vi "File taratura assente.vi"(8 "Curva 3":string[][](array[string]), 9 "Curva 2":string[][](array[string]), 10 "Curva 1":string[][](array[string]), 11 "P2":i32) -> (2 "File taratura assente":bool)   [LabVIEW 2019]
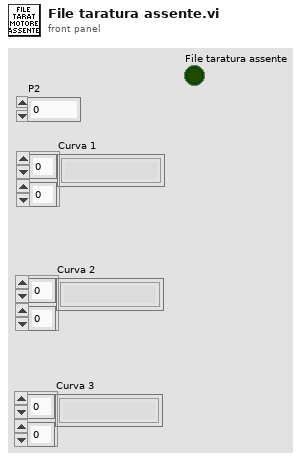
[diagram p1: front panel]
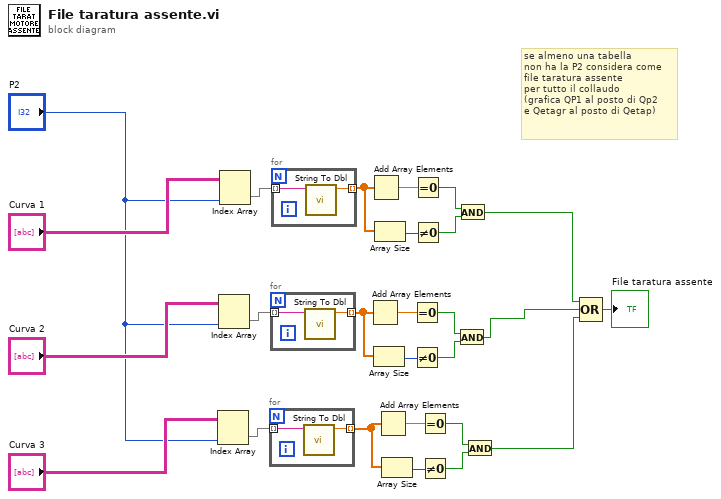
[diagram p0: block diagram]
diagram:
  # "se almeno una tabella\nnon ha la P2 considera come\nfile taratura assente \nper tutto il collaudo \n(grafica QP1 al posto di Qp2\ne Qetagr al posto di Qetap)"
  n1 = Index Array(array="Curva 3", index (col)="P2") -> (element=w21:string[])  [unwired: 1 in]
  n2 = Index Array(array="Curva 2", index (col)="P2") -> (element=w22:string[])  [unwired: 1 in]
  n3 = Index Array(array="Curva 1", index (col)="P2") -> (element=w25:string[])  [unwired: 1 in]
  n4 = for {
    tunnel: w21 -> [w28] mode=indexing
    tunnel: [w27] -> w5 mode=indexing
    n5 = call "String To Dbl.vi"("String"=w28) -> ("Numeric"=w27:dbl)  [unwired: 10 in]
  }
  n6 = for {
    tunnel: w22 -> [w30] mode=indexing
    tunnel: [w29] -> w10 mode=indexing
    n7 = call "String To Dbl.vi"("String"=w30) -> ("Numeric"=w29:dbl)  [unwired: 10 in]
  }
  n8 = for {
    tunnel: w25 -> [w32] mode=indexing
    tunnel: [w31] -> w18 mode=indexing
    n9 = call "String To Dbl.vi"("String"=w32) -> ("Numeric"=w31:dbl)  [unwired: 10 in]
  }
  n10 = Add Array Elements(numeric array=w10) -> (sum=w11:dbl)
  n11 = Add Array Elements(numeric array=w18) -> (sum=w26:dbl)
  n12 = Array Size(array=w10) -> (size(s)=w12:i32)
  n13 = Array Size(array=w18) -> (size(s)=w17:i32)
  n14 = Add Array Elements(numeric array=w5) -> (sum=w9:dbl)
  n15 = Array Size(array=w5) -> (size(s)=w8:i32)
  n16 = Equal To 0?(x=w11) -> (x = 0?=w14:bool)
  n17 = Not Equal To 0?(x=w12) -> (x != 0?=w13:bool)
  n18 = Equal To 0?(x=w26) -> (x = 0?=w15:bool)
  n19 = Not Equal To 0?(x=w17) -> (x != 0?=w16:bool)
  n20 = Equal To 0?(x=w9) -> (x = 0?=w6:bool)
  n21 = Not Equal To 0?(x=w8) -> (x != 0?=w7:bool)
  n22 = And(x=w14, y=w13) -> (x .and. y?=w3:bool)
  n23 = And(x=w15, y=w16) -> (x .and. y?=w4:bool)
  n24 = And(x=w6, y=w7) -> (x .and. y?=w2:bool)
  n25 = Compound Arithmetic op=OR(w4, w3, w2) -> (→"File taratura assente":bool)
